vi "DEMO Read Sequence.vi"() -> ()   [LabVIEW 2017]
uses:
  SequenceSubvis/TestStep-StepType.ctl
  SequenceSubvis/RF Direction.ctl
  SequenceSubvis/PolarizationSelect.ctl
  SequenceSubvis/TestStepTypes.ctl
  Sequence.lvclass
  seqConfig.ctl
panel:
  out "error out":errorcluster
  out "TestSequence":T1[](array[typedef])
  in  "Path":path=path "C:/Users/Public/Documents/UCAR/APAR Board Test/SupportFiles/aparTempSequence.xml"
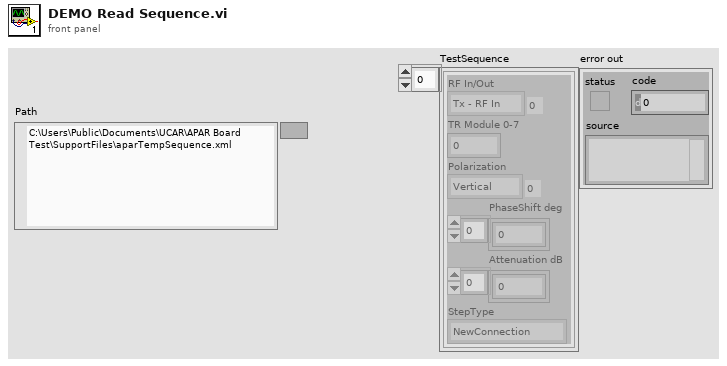
[diagram p1: front panel]
types:
  T1 = typedef "TestStep-StepType.ctl" = cluster{"RF In/Out":T2, "TR Module 0-7":i32, "Polarization":T3, "PhaseShift deg":dbl[], "Attenuation dB":dbl[], "StepType":T4}
  T2 = typedef "RF Direction.ctl" = enum16{"Tx - RF In", "Rx - RF Out"}
  T3 = typedef "PolarizationSelect.ctl" = enum16{"Vertical", "Horizontal"}
  T4 = typedef "TestStepTypes.ctl" = enum16{"NewConnection", "SweepTest", "Motion", "Finish"}
  T5 = typedef "seqConfig.ctl" = cluster{"TempXMLFilePath":path, "Motion":bool}
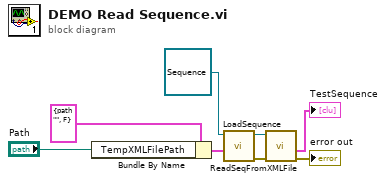
[diagram p0: block diagram]
diagram:
  n1 = Bundle By Name(cluster=T5 {"TempXMLFilePath"=path "", "Motion"=FALSE} ("Sequence Cfg"), "TempXMLFilePath"="Path") -> (w4:T5)
  n2 = call "LoadSequence.vi"("Sequence Cfg"=w4, "Sequence in"=refnum<class "Sequence.lvclass"> refnum) -> ("error out"=w3:errorcluster, "Sequence out"=w8:refnum<class "Sequence.lvclass">)  [unwired: 8 in]
  n3 = call "ReadSeqFromXMLFile.vi"("error in (no error)"=w3, "Sequence in"=w8) -> ("error out"=→"error out":errorcluster, "TestSequence"=→"TestSequence":T1[])  [unwired: 6 in, 2 out]
